vi "lvBuild.vi"(8 "error in (no error)":errorcluster, 11 "CommandLine":string[](array[string])) -> (0 "error out":errorcluster, 2 "test details":string)   [LabVIEW 2019]
uses:
  <vilib>/AppBuilder/AB_API_Simple/Build (path).vi
  <vilib>/AppBuilder/AB_API_Simple/NI_App_Builder_API.lvlib
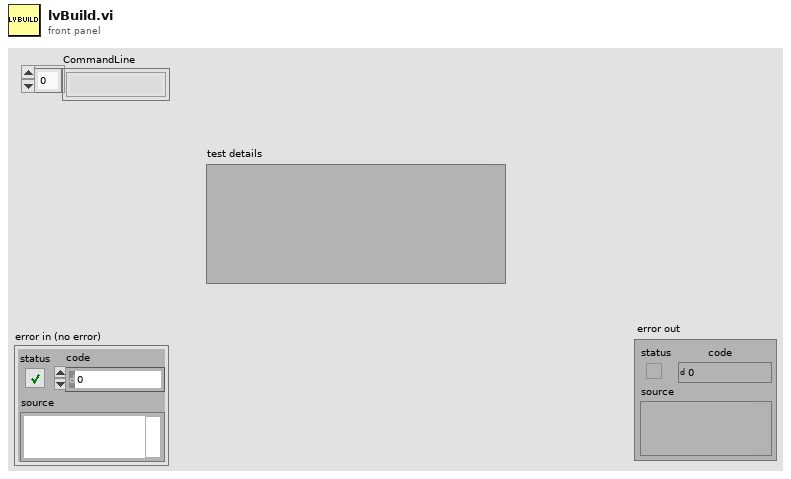
[diagram p1: front panel]
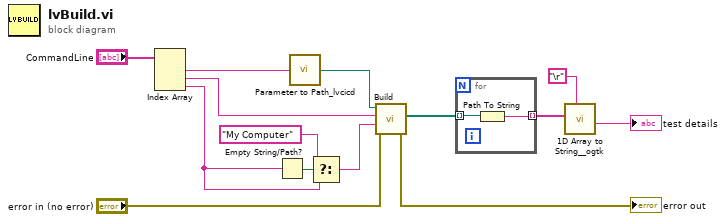
[diagram p0: block diagram]
diagram:
  n1 = Index Array(array="CommandLine") -> (element #1=w5:string, element #2=w11:string, element #3=w2:string)  [unwired: 3 in]
  n2 = Empty String/Path?(string/path=w2) -> (empty?=w4:bool)
  n3 = call "Parameter to Path_lvcicd.vi"("String"=w5) -> ("Path"=w6:path)
  n4 = Select(t="My Computer" ("element"), s=w4, f=w2) -> (s? t:f=w1:string)
  n5 = call-poly <vilib>:"Build.vi"("error in (no error)"="error in (no error)", "Name of target (My Computer)"=w1, "Name of build specification (if empty: build all)"=w11, "Path to project"=w6) -> ("error out"=→"error out":errorcluster, "Generated files"=w10:path[])  [unwired: 6 in]
  n6 = for {
    tunnel: w10 -> [w16] mode=indexing
    tunnel: [w15] -> w9 mode=indexing
    n7 = Path To String(path=w16) -> (string=w15:string)
  }
  n8 = call <userlib>:"1D Array to String__ogtk.vi"("delimiter (Tab)"="\r", "Array of Strings"=w9) -> ("delimited string"=→"test details":string)  [unwired: 9 in]
